vi "ProgramStatusFGV.vi"(0 "Application Interface in":refnum<class "Application Interface.lvclass">, 1 "Program Status":T1, 5 "error in (no error)":errorcluster, 9 "Action (Read)":T3=enum."Get Last Status") -> (14 "Application Interface out":refnum<class "Application Interface.lvclass">, 15 "Program Status out":T1, 19 "error out":errorcluster)   [LabVIEW 2016, in "Application Interface.lvclass"]
uses:
  Application Interface.lvclass
  FGVAction.ctl
  Robot/Universal Robot/ProgramStatus.ctl
  Robot/Universal Robot/ProgramState.ctl
  Robot/Universal Robot/Universal Robot.lvclass
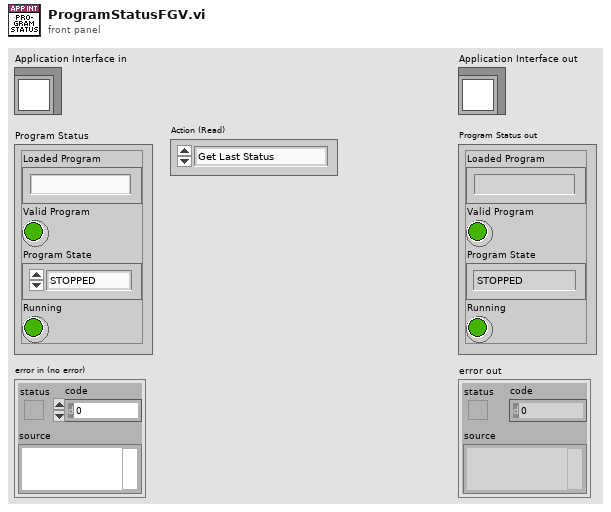
[diagram p1: front panel]
types:
  T1 = typedef "Universal Robot.lvclass/ProgramStatus.ctl" = cluster{"Loaded Program":string, "Valid Program":bool, "Program State":T2, "Running":bool}
  T2 = typedef "Universal Robot.lvclass/ProgramState.ctl" = enum16{"STOPPED", "PLAYING", "PAUSE"}
  T3 = typedef "Application Interface.lvclass/FGVAction.ctl" = enum16{"Initialize", "Get Last Status", "Update Status"}
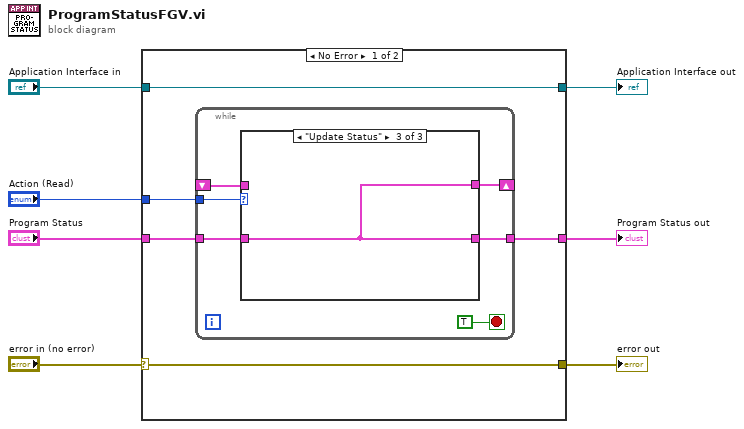
[diagram p0: block diagram]
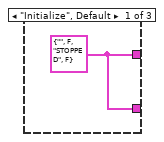
[diagram p2: hidden frame]
diagram:
  n1 = case shown="No Error" "error in (no error)" {
    selector: "error in (no error)" -> [w8 w23]
    tunnel: [w8 w23] -> w6
    tunnel: [w12 w22] -> w4
    tunnel: "Application Interface in" -> [w12 w22]
    tunnel: "Program Status" -> [w11 _]
    tunnel: "Action (Read)" -> [w10 _]
    tunnel: [w9 _] -> w1
    frame No Error {
      n2 = while {
        tunnel: w11 -> [w17]
        tunnel: w10 -> [w16]
        shift-right: [w15] -> _
        shift-left: _ -> [w14]
        tunnel: [w13] -> w9
        stop <- TRUE stop-if-true
        n3 = case shown="\"Update Status\"" w16 {
          tunnel: w17 -> [_ _ w21]
          tunnel: [w19 w20 w21] -> w15
          tunnel: w14 -> [_ w20 _]
          tunnel: [w19 w20 w21] -> w13
          frame "Initialize", Default {
            w19 = T1 {"Loaded Program"="", "Valid Program"=FALSE, "Program State"=enum."STOPPED", "Running"=FALSE} ("Program Status")
          }
          frame "Get Last Status" {
          }
          frame "Update Status" {
          }
        }
      }
    }
    frame Error {
    }
  }
  "error out" <- w6
  "Application Interface out" <- w4
  "Program Status out" <- w1
